vi "Get Intensity Color.vi"(11 "Color Ramp Cluster":T1={"Color Ramp Style"=enum."None", "Color Ramp Array"=[16711934, 393471, 57855, 4390754, 16449346, 16744722, 16711680], "Color Ramp Index"=[45, 91, 133, 175, 219, 255], "Interpolate?"=FALSE, "Logarithm?"=FALSE}) -> (3 "Intensity Color":u32[](array[numeric]))   [LabVIEW 2020, in "3D Plot.lvclass"]
uses:
  3D Plot.lvclass
  Color Ramp Cluster.ctl
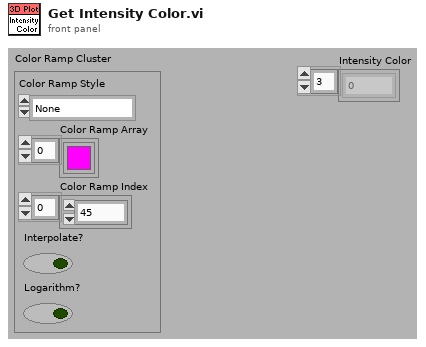
[diagram p1: front panel]
types:
  T1 = typedef "3D Plot.lvclass/Color Ramp Cluster.ctl" = cluster{"Color Ramp Style":enum16{"None", "Shaded", "Color spectrum", "Grey scale", "Custom"}, "Color Ramp Array":u32[], "Color Ramp Index":i32[], "Interpolate?":bool, "Logarithm?":bool}
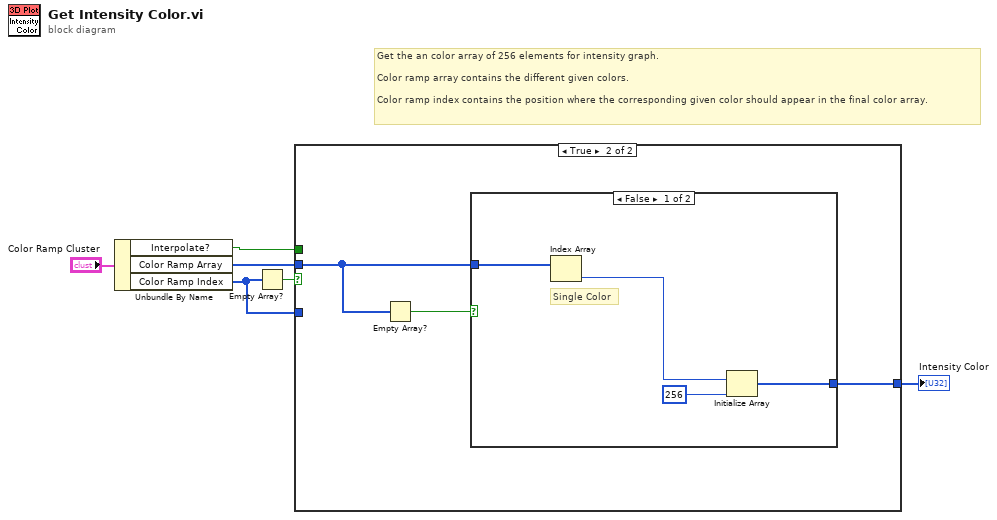
[diagram p0: block diagram]
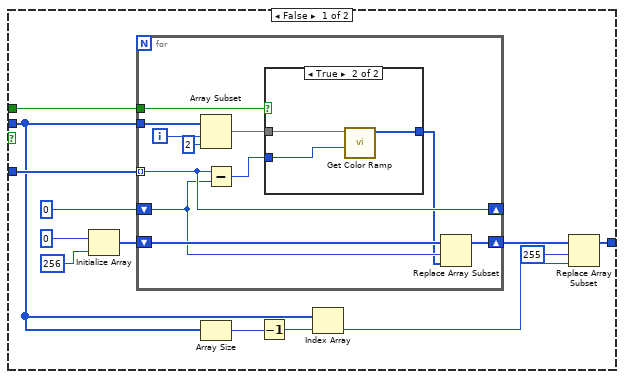
[diagram p2: hidden frame]
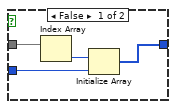
[diagram p3: hidden frame]
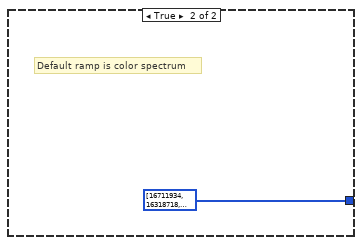
[diagram p4: hidden frame]
diagram:
  # "Get the an color array of 256 elements for intensity graph.\n\nColor ramp array contains the different given colors.\n\nColor ramp index contains the position where the corresponding given color should appear in the final color array."
  n1 = Unbundle By Name("Color Ramp Cluster") -> ("Interpolate?"=w1:bool, "Color Ramp Array"=w3:u32[], "Color Ramp Index"=w2:i32[])
  n2 = Empty Array?(array=w2) -> (empty?=w5:bool)
  n3 = case shown="True" w5 {
    tunnel: w2 -> [w15 _]
    tunnel: w1 -> [w14 _]
    tunnel: [w12 w40] -> w6
    tunnel: w3 -> [w9 w39]
    frame False {
      n4 = Initialize Array(u32 0, 256 ("dimension size")) -> (w18:u32[])
      n5 = for {
        tunnel: w15 -> [w26] mode=indexing
        tunnel: w9 -> [w30]
        shift-right: [w26] -> _
        shift-left: 0 ("Numeric 4") -> [w23]
        shift-right: [w24] -> w13
        shift-left: w18 -> [w25]
        tunnel: w14 -> [w20]
        i -> [w29]
        n6 = Array Subset(array=w30, index=w29, length=2) -> (w27:u32[])
        n7 = Subtract(x=w26, y=w23) -> (x-y=w22:i32)
        n8 = case shown="True" w20 {
          tunnel: w27 -> [w33 w37]
          tunnel: w22 -> [w34 w36]
          tunnel: [w31 w35] -> w21
          frame False {
            n9 = Index Array(array=w33) -> (element=w32:u32)  [unwired: 1 in]
            n10 = Initialize Array(w32, w34) -> (w31:u32[])
          }
          frame True {
            n11 = call "Get Color Ramp.vi"("Number of Colors"=w36, "Color Ramp Array"=w37) -> ("RGB Array"=w35:u32[])  [unwired: 9 out]
          }
        }
        n12 = Replace Array Subset(array=w25, new element=w21, index=w23) -> (w24:u32[])
      }
      n13 = Array Size(array=w9) -> (size(s)=w11:i32)
      n14 = Decrement(x=w11) -> (x-1=w10:i32)
      n15 = Index Array(array=w9, index=w10) -> (element=w8:u32)
      n16 = Replace Array Subset(array=w13, new element=w8, index=255) -> (w12:u32[])
    }
    frame True {
      n17 = Empty Array?(array=w39) -> (empty?=w38:bool)
      n18 = case shown="False" w38 {
        tunnel: [w42 u32[] [16711934, 16318718, 15925502, 15597822, 15204606, 14876926, 14483710, 14156030, 13762814, 13435134, 13041918, 12714238, 12321022, 11993342, 11600126, 11272446, 10879230, 10486014, 10158334, 9765118, 9437438, 9044222, 8716542, 8323326, 7995646, 7602430, 7274750, 6881534, 6553854, 6160638, 5832958, 5439742, 5046526, 4718846, 4325630, 3997950, 3604734, 3277054, 2883838, 2556158, 2162942, 1835262, 1442046, 1114366, 721150, 393471, 328959, 330239, 331519, 332799, 334079, 335359, 336639, 272383, 273663, 274687, 275967, 277247, 278527, 279807, 281087, 216831, 218111, 219391, 220415, 221695, 222975, 224255, 225535, 161279, 162559, 163839, 165119, 166143, 167423, 168703, 104447, 105727, 107007, 108287, 109567, 110847, 111871, 113151, 48895, 50175, 51455, 52735, 54015, 55295, 56575, 57855, 123387, 254711, 320499, 451568, 517356, 648680, 780004, 845537, 976861, 1042649, 1173717, 1239506, 1370830, 1502154, 1567686, 1699011, 1764799, 1895867, 1961655, 2092980, 2224304, 2289836, 2421161, 2486949, 2618017, 2683805, 2815130, 2946454, 3011986, 3143310, 3209099, 3340167, 3405955, 3537279, 3668604, 3734136, 3865460, 3931248, 4062317, 4128105, 4259429, 4390754, 4652897, 4915040, 5242719, 5504862, 5767006, 6094685, 6356828, 6684507, 6946651, 7208794, 7536473, 7798616, 8060760, 8388439, 8650582, 8978261, 9240405, 9502548, 9830227, 10092370, 10420050, 10682193, 10944336, 11272015, 11534158, 11796302, 12123981, 12386124, 12713803, 12975947, 13238090, 13565769, 13827912, 14090056, 14417735, 14679878, 15007557, 15269701, 15531844, 15859523, 16121666, 16449346, 16448576, 16447807, 16447038, 16446269, 16445500, 16444731, 16443962, 16443449, 16508216, 16507447, 16506678, 16505908, 16505139, 16504370, 16503857, 16503088, 16502319, 16567086, 16566317, 16565548, 16564779, 16564266, 16563496, 16562727, 16561958, 16561189, 16625956, 16625187, 16624418, 16623905, 16623136, 16622367, 16621598, 16620828, 16620059, 16684826, 16684313, 16683544, 16682775, 16682006, 16681237, 16680468, 16679699, 16744722, 16743697, 16742673, 16741904, 16740880, 16740111, 16739087, 16738062, 16737294, 16736269, 16735501, 16734476, 16733708, 16732683, 16731659, 16730890, 16729866, 16729097, 16728073, 16727048, 16726280, 16725255, 16724486, 16723462, 16722694, 16721669, 16720645, 16719876, 16718852, 16718083, 16717058, 16716034, 16715266, 16714241, 16713473, 16712448, 16711680] ("Intensity Color 2")] -> w40
        tunnel: w39 -> [w41 _]
        frame False {
          # "Single Color"
          n19 = Index Array(array=w41) -> (element=w44:u32)  [unwired: 1 in]
          n20 = Initialize Array(w44, 256 ("dimension size")) -> (w42:u32[])
        }
        frame True {
          # "Default ramp is color spectrum"
        }
      }
    }
  }
  "Intensity Color" <- w6
